vi "MH_InsertIntoTimeTrace.vi"(6 "TimeTrace in":u32[][](array[numeric]), 8 "NumVals":i32, 9 "Vals":u32[][](array[numeric]), 10 "LengthTTrace":u64, 11 "TimeTraceBin":i32) -> (3 "TimeTrace out":u32[][](array[numeric]))   [LabVIEW 2010]
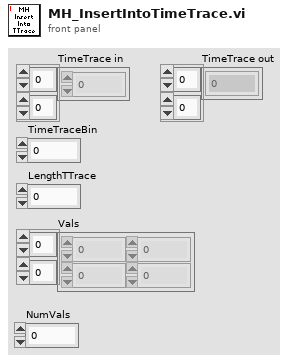
[diagram p1: front panel]
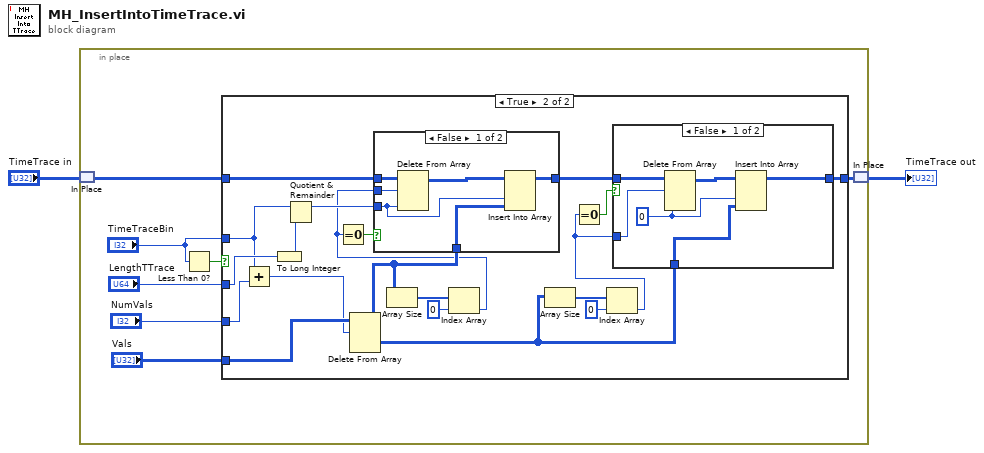
[diagram p0: block diagram]
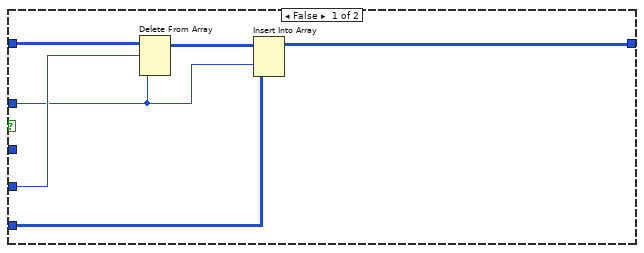
[diagram p2: hidden frame]
diagram:
  n1 = in-place {
    n2 = in-place-match #1("TimeTrace in") -> (w4:u32[][])
    n3 = Less Than 0?(x="TimeTraceBin") -> (x < 0?=w6:bool)
    n4 = case shown="True" w6 {
      tunnel: w4 -> [w15 w35]
      tunnel: "Vals" -> [w12 w33]
      tunnel: [w10 w34] -> w3
      tunnel: "TimeTraceBin" -> [w11 w30]
      tunnel: "LengthTTrace" -> [_ w32]
      tunnel: "NumVals" -> [w14 w31]
      frame False {
        n5 = Delete From Array(array=w15, length=w14, index (col)=w11) -> (array with subset deleted=w13:u32[][])  [unwired: 1 in, 1 out]
        n6 = Insert Into Array(array=w13, index (col)=w11, new element=w12) -> (w10:u32[][])  [unwired: 1 in]
      }
      frame True {
        n7 = Add(x=w30, y=w31) -> (x+y=w29:i32)
        n8 = To Long Integer(number=w32) -> (32bit integer=w28:i32)
        n9 = Quotient & Remainder(x=w30, y=w28) -> (x-y*floor(x/y)=w27:i32)  [unwired: 1 out]
        n10 = Delete From Array(array=w33, length=w29) -> (deleted portion=w20:u32[][], array with subset deleted=w25:u32[][])  [unwired: 2 in]
        n11 = Array Size(array=w25) -> (size(s)=w24:i32[])
        n12 = Index Array(array=w24, index=0) -> (element=w17:i32)
        n13 = Equal To 0?(x=w17) -> (x = 0?=w19:bool)
        n14 = case shown="False" w19 {
          tunnel: w35 -> [w47 w49]
          tunnel: w27 -> [w43 _]
          tunnel: [w46 w49] -> w26
          tunnel: w25 -> [w45 _]
          tunnel: w17 -> [w44 _]
          frame False {
            n15 = Delete From Array(array=w47, length=w44, index (col)=w43) -> (array with subset deleted=w48:u32[][])  [unwired: 1 in, 1 out]
            n16 = Insert Into Array(array=w48, index (col)=w43, new element=w45) -> (w46:u32[][])  [unwired: 1 in]
          }
          frame True {
          }
        }
        n17 = Array Size(array=w20) -> (size(s)=w21:i32[])
        n18 = Index Array(array=w21, index=0) -> (element=w16:i32)
        n19 = Equal To 0?(x=w16) -> (x = 0?=w18:bool)
        n20 = case shown="False" w18 {
          tunnel: [w38 w42] -> w34
          tunnel: w26 -> [w40 w42]
          tunnel: w20 -> [w37 _]
          tunnel: w16 -> [w41 _]
          frame False {
            w36 = 0 ("disabled index (col)")
            n21 = Delete From Array(array=w40, length=w41, index (col)=w36) -> (array with subset deleted=w39:u32[][])  [unwired: 1 in, 1 out]
            n22 = Insert Into Array(array=w39, index (col)=w36, new element=w37) -> (w38:u32[][])  [unwired: 1 in]
          }
          frame True {
          }
        }
      }
    }
    n23 = in-place-match #1(w3) -> (→"TimeTrace out":u32[][])
  }
